vi "FoundInstruments.vi"(8 "error in (no error)":errorcluster, 10 "Instruments Found":T1, 11 "InitDeinitComm in":refnum<class "InitDeinitComm.lvclass">) -> (0 "error out":errorcluster, 3 "InitDeinitComm out":refnum<class "InitDeinitComm.lvclass">)   [LabVIEW 2023, in "InitDeInit.lvlib" / "InitDeinitComm.lvclass"]
uses:
  InitDeinitComm.lvclass
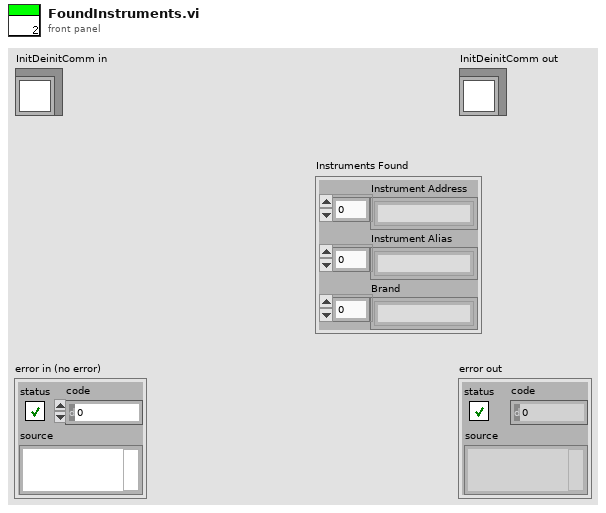
[diagram p1: front panel]
types:
  T1 = cluster{"Instrument Address":string[], "Instrument Alias":string[], "Brand":string[]}
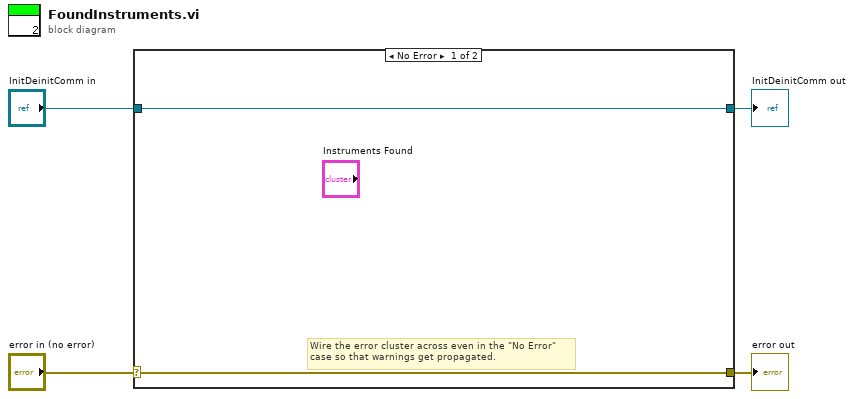
[diagram p0: block diagram]
diagram:
  n1 = case shown="No Error" "error in (no error)" {
    selector: "error in (no error)" -> [w5 w8]
    tunnel: [w5 w8] -> w3
    tunnel: [w6 w7] -> w1
    tunnel: "InitDeinitComm in" -> [w6 w7]
    frame No Error {
      # "Wire the error cluster across even in the \"No Error\"\ncase so that warnings get propagated."
    }
    frame Error {
    }
  }
  "error out" <- w3
  "InitDeinitComm out" <- w1
